vi "Read DUT Info.vi"(8 "error in (no error)":errorcluster, 11 "Execution in":refnum<class "Execution.lvclass">) -> (0 "error out":errorcluster, 2 "DUT Info":T1, 3 "Execution out":refnum<class "Execution.lvclass">)   [LabVIEW 2015, in "Execution.lvclass"]
uses:
  Execution.lvclass
  DUT_INFO_TYPEDEF.ctl
  Execution.lvclass/Execution.ctl
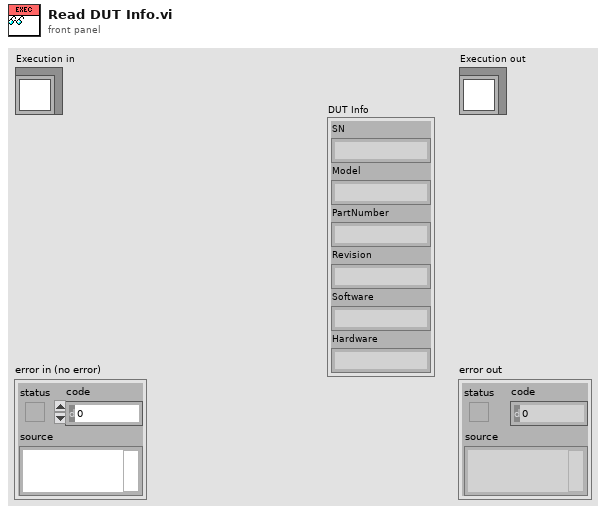
[diagram p1: front panel]
types:
  T1 = typedef "Execution.lvclass/DUT_INFO_TYPEDEF.ctl" = cluster{"SN":string, "Model":string, "PartNumber":string, "Revision":string, "Software":string, "Hardware":string}
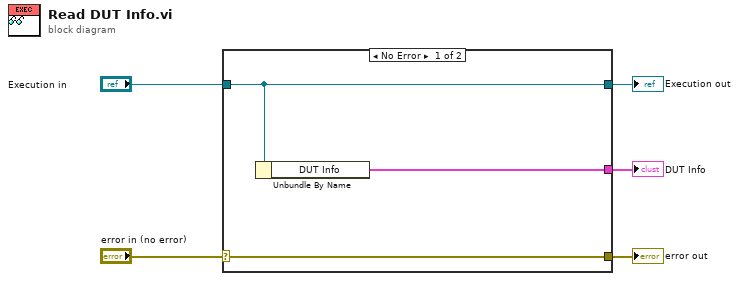
[diagram p0: block diagram]
diagram:
  n1 = case shown="No Error" "error in (no error)" {
    selector: "error in (no error)" -> [w8 w9]
    tunnel: [w8 w9] -> w4
    tunnel: [w7 w10] -> w2
    tunnel: "Execution in" -> [w7 w10]
    tunnel: [w6 _] -> w1
    frame No Error {
      n2 = Unbundle By Name(w7) -> ("DUT Info"=w6:T1)
    }
    frame Error {
    }
  }
  "error out" <- w4
  "Execution out" <- w2
  "DUT Info" <- w1
